vi "Teleop.vi"(10 "Match Info":T1={"Autonomous Elapsed Seconds"=0.0, "TeleOp Elapsed Seconds"=0.0, "Disabled Elapsed Seconds"=0.0, "Visited Autonomous"=FALSE, "Visited TeleOp"=FALSE, "Visited Disabled"=FALSE, "Autonomous Settings"={"Autonomous Style"=enum."Independent", "VI Refnum"=refnum}}, 11 "Call Context":T2) -> ()   [LabVIEW 2014]
doc: "This VI is called for each TeleOp packet received from the DS where the robot is not disabled. It is often used to read from the joysticks and update I/O or to update setpoints for timed control loops. It should complete and return within 20 milliseconds or it may miss DS packets."
uses:
  <vilib>/Rock Robotics/WPI/DriverStation/WPI_DriverStationDerivedRobotMode.ctl
  <vilib>/Rock Robotics/WPI/DriverStation/WPI_DriverStationMatch Info.ctl
  <vilib>/Rock Robotics/WPI/RobotDrive/WPI_RobotDriveGetSetRefNum.vi
  <vilib>/Rock Robotics/WPI/Joystick/WPI_JoystickGetSetRefNum.vi
  <vilib>/Rock Robotics/Network Tables/SD Write Boolean Array.vi
  <vilib>/Rock Robotics/Network Tables/SD Write Numeric Array.vi
  <vilib>/Rock Robotics/Network Tables/SD Read Boolean.vi
  <vilib>/Rock Robotics/Network Tables/SD Read Number.vi
  <vilib>/Rock Robotics/WPI/RobotDrive/WPI_RobotDriveMecanumDrive_Cartesian.vi
panel:
  out "Elevator At Middle":bool
  out "Linear Debug":dbl
  out "Debug":dbl format="%#_13g"
  out "Elevator Up":bool=TRUE
  out "Elevator Down":bool=TRUE
  out "Sample Slider 0":dbl(slide) scale=0.0..5.0
  out "Sample Boolean 1":bool
  out "Sample Boolean 0":bool
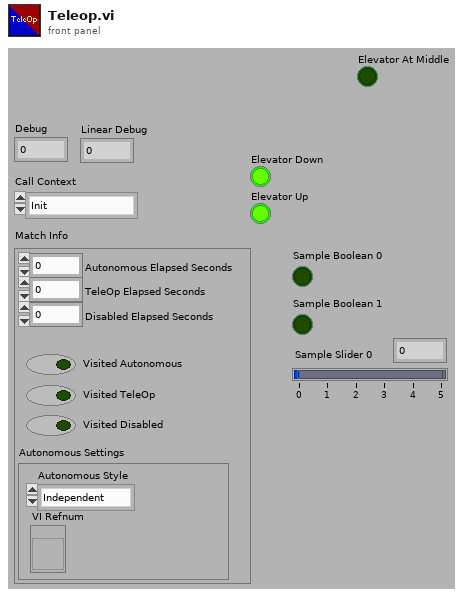
[diagram p1: front panel]
types:
  T1 = typedef "WPI_DriverStationMatch Info.ctl" = cluster{"Autonomous Elapsed Seconds":dbl, "TeleOp Elapsed Seconds":dbl, "Disabled Elapsed Seconds":dbl, "Visited Autonomous":bool, "Visited TeleOp":bool, "Visited Disabled":bool, "Autonomous Settings":cluster{"Autonomous Style":enum16{"Iterative", "Independent"}, "VI Refnum":refnum<vi>}}
  T2 = typedef "WPI_DriverStationDerivedRobotMode.ctl" = enum16{"Init", "Execute", "Stop"}
  T3 = typedef "WPI_RobotDriveDevRef.ctl" = cluster{"DevStatus":errorcluster, "Motors[]":T4[], "Square Inputs":bool, "Max Output":dbl}
  T4 = typedef "WPI_MotorControlDeviceRef.ctl" = cluster{"DeviceStatus":errorcluster, "Type":T5, "PWM":cluster{"Controller":T6, "PWM Channel":T7, "DeadBand":T8}, "CAN":cluster{"Device Number":u8, "Control Mode":T9, "Semaphore":T10, "Max Vout":dbl, "TalonSRX Control Mode":T11}, "Invert":bool, "TransformRef":T12, "InvTransformRef":T12}
  T5 = typedef "WPI_MotorControlType.ctl" = enum16{"PWM", "CAN", "CANTalonSRX"}
  T6 = typedef "FPGA_TypedefDigitalModule.ctl" = enum16{"Controller 1"}
  T7 = typedef "FPGA_DIOPWMChannel.ctl" = enum8{"PWM 0", "PWM 1", "PWM 2", "PWM 3", "PWM 4", "PWM 5", "PWM 6", "PWM 7", "PWM 8", "PWM 9", "PWM MXP 0", "PWM MXP 1", "PWM MXP 2", "PWM MXP 3", "PWM MXP 4", "PWM MXP 5", "PWM MXP 6", "PWM MXP 7", "PWM MXP 8", "PWM MXP 9", "Invalid"}
  T8 = typedef "WPI_PWMDeadband.ctl" = cluster{"Name":string, "maxPositivePwm":i32, "minPositivePwm":i32, "centerPwm":i32, "maxNegativePwm":i32, "minNegativePwm":i32, "angularRange":u16}
  T9 = typedef "WPI_CANJaguar_ControlMode.ctl" = enum8{"Percent VBus", "Current", "Speed", "Position", "Voltage"}
  T10 = typedef "Semaphore RefNum" = refnum<k1>
  T11 = typedef "WPI_CANTalonSRX_APIControlMode.ctl" = enum8{"Percent VBus", "Speed", "Position", "Slave", "Unchanged / Invalid"}
  T12 = typedef "WPI_PWMTransform_ConPane.ctl" = refnum<vi>
  T13 = typedef "WPI_JoystickDevRef.ctl" = cluster{"Device":T14}
  T14 = typedef "WPI_JoystickDeviceEnum.ctl" = enum16{"USB 0", "USB 1", "USB 2", "USB 3", "USB 4", "USB 5"}
  T15 = typedef "WPI_DigitalInputDevRef.ctl" = cluster{"DevStatus":errorcluster, "DIO Channel":T16, "Controller":T6}
  T16 = typedef "FPGA_DIOChannel.ctl" = enum8{"DIO 0", "DIO 1", "DIO 2", "DIO 3", "DIO 4", "DIO 5", "DIO 6", "DIO 7", "DIO 8", "DIO 9", "DIO MXP 0", "DIO MXP 1", "DIO MXP 2", "DIO MXP 3", "DIO MXP 4", "DIO MXP 5", "DIO MXP 6", "DIO MXP 7", "DIO MXP 8", "DIO MXP 9", "DIO MXP 10", "DIO MXP 11", "DIO MXP 12", "DIO MXP 13", "DIO MXP 14", "DIO MXP 15", "Invalid"}
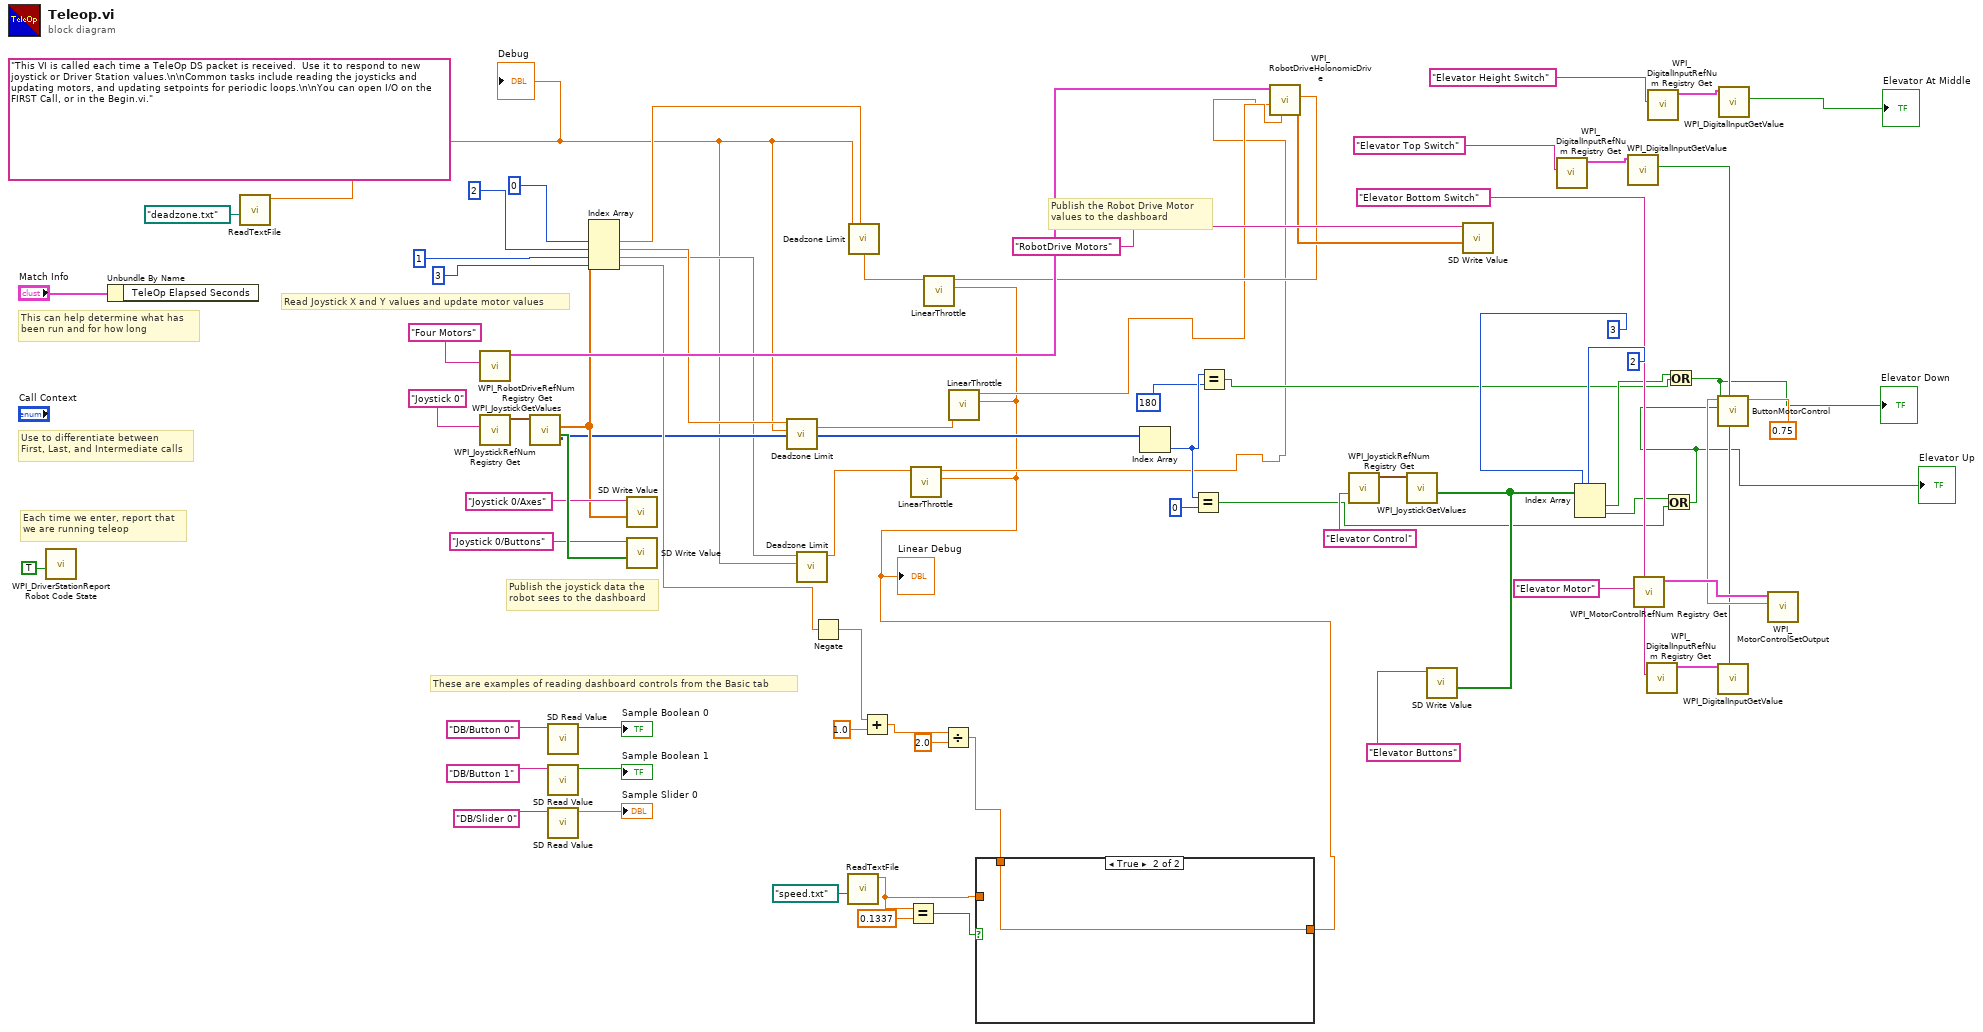
[diagram p0: block diagram]
diagram:
  (unwired) "This VI is called each time a TeleOp DS packet is received.  Use it to respond to new joystick or Driver Station values.\n\nCommon tasks include reading the joysticks and updating motors, and updating setpoints for periodic loops.\n\nYou can open I/O on the FIRST Call, or in the Begin.vi."
  # "These are examples of reading dashboard controls from the Basic tab"
  # "Publish the Robot Drive Motor\nvalues to the dashboard"
  # "Publish the joystick data the\nrobot sees to the dashboard"
  # "Each time we enter, report that\nwe are running teleop"
  # "Use to differentiate between\nFirst, Last, and Intermediate calls"
  # "This can help determine what has\nbeen run and for how long"
  # "Read Joystick X and Y values and update motor values"
  n1 = call <vilib>:"WPI_DriverStationReport Robot Code State.vi"("TeleOp"=TRUE ("Autonomous")) -> ()  [unwired: 10 in, 1 out]
  n2 = Unbundle By Name("Match Info") -> ()  [unwired: 1 out]
  n3 = call "ReadTextFile.vi"("file (use dialog)"=path "/deadzone.txt") -> ("Double"=w7:dbl)  [unwired: 9 in, 1 out]
  "Debug" <- w7
  n4 = call <vilib>:"WPI_RobotDriveRefNum Registry Get.vi"("refnum name"="Four Motors") -> ("RobotDriveDevRef"=w71:T3)  [unwired: 1 in, 9 out]
  n5 = call <vilib>:"WPI_JoystickRefNum Registry Get.vi"("refnum name"="Joystick 0") -> ("JoystickDevRef"=w69:T13)  [unwired: 1 in, 9 out]
  n6 = call <vilib>:"WPI_JoystickGetValues.vi"("JoystickDevRef"=w69) -> ("Buttons"=w67:bool[], "Axes"=w56:dbl[], "POVs"=w28:i16[])  [unwired: 6 in, 2 out]
  n7 = call-poly <vilib>:"SD Read Value.vi"("Name"="DB/Button 0" ("refnum name")) -> ("Boolean"=→"Sample Boolean 0":bool)  [unwired: 8 in, 2 out]
  n8 = call-poly <vilib>:"SD Read Value.vi"("Name"="DB/Button 1" ("refnum name")) -> ("Boolean"=→"Sample Boolean 1":bool)  [unwired: 8 in, 2 out]
  n9 = call-poly <vilib>:"SD Read Value.vi"("Name"="DB/Slider 0" ("refnum name")) -> ("Numeric"=→"Sample Slider 0":dbl)  [unwired: 8 in, 2 out]
  n10 = Index Array(array=w56, index #1=0 ("X"), index #2=2 ("Y"), index #3=1 ("Rotate"), index #4=3 ("throttle")) -> (element #1=w47:dbl, element #2=w46:dbl, element #3=w15:dbl, element #4=w38:dbl)
  n11 = call-poly <vilib>:"SD Write Value.vi"("Numeric Array"=w56, "Name"="Joystick 0/Axes") -> ()  [unwired: 8 in, 2 out]
  n12 = call-poly <vilib>:"SD Write Value.vi"("Boolean Array"=w67, "Name"="Joystick 0/Buttons") -> ()  [unwired: 8 in, 2 out]
  n13 = call "Deadzone Limit.vi"("Limit"=w7, "Input"=w46) -> ("Output"=w41:dbl)  [unwired: 9 in]
  n14 = call "Deadzone Limit.vi"("Limit"=w7, "Input"=w15) -> ("Output"=w40:dbl)  [unwired: 9 in]
  n15 = Negate(x=w38) -> (-x=w39:dbl)
  n16 = call "ReadTextFile.vi"("file (use dialog)"=path "/speed.txt") -> ("Double"=w1:dbl)  [unwired: 9 in, 1 out]
  n17 = call "Deadzone Limit.vi"("Limit"=w7, "Input"=w47) -> ("Output"=w42:dbl)  [unwired: 9 in]
  n18 = Add(x=w39, y=1.0) -> (x+y=w44:dbl)
  n19 = Equal?(x=w1, y=0.1337) -> (x = y?=w4:bool)
  n20 = Divide(x=w44, y=2.0) -> (x/y=w3:dbl)
  n21 = case shown="True" w4 {
    tunnel: w3 -> [_ w75]
    tunnel: [w74 w75] -> w2
    tunnel: w1 -> [w74 _]
    frame False {
    }
    frame True {
    }
  }
  "Linear Debug" <- w2
  n22 = call "LinearThrottle.vi"("Throttle"=w2, "Value"=w40) -> ("Numeric"=w9:dbl)  [unwired: 9 in]
  n23 = call "LinearThrottle.vi"("Throttle"=w2, "Value"=w42) -> ("Numeric"=w37:dbl)  [unwired: 9 in]
  n24 = call "LinearThrottle.vi"("Throttle"=w2, "Value"=w41) -> ("Numeric"=w10:dbl)  [unwired: 9 in]
  n25 = Index Array(array=w28) -> (element=w24:i16)  [unwired: 1 in]
  n26 = Equal?(x=w24, y=i16 0) -> (x = y?=w18:bool)
  n27 = Equal?(x=w24, y=i16 180) -> (x = y?=w19:bool)
  n28 = call-poly <vilib>:"WPI_RobotDriveHolonomicDrive.vi"("Rotation"=w10, "Y"=w9, "X"=w37, "RobotDriveDevRef"=w71) -> ("Motor Values"=w57:dbl[])  [unwired: 5 in, 2 out]
  n29 = call <vilib>:"WPI_JoystickRefNum Registry Get.vi"("refnum name"="Elevator Control") -> ("JoystickDevRef"=w54:T13)  [unwired: 1 in, 9 out]
  n30 = call <vilib>:"WPI_JoystickGetValues.vi"("JoystickDevRef"=w54) -> ("Buttons"=w52:bool[])  [unwired: 6 in, 4 out]
  n31 = call-poly <vilib>:"SD Write Value.vi"("Boolean Array"=w52, "Name"="Elevator Buttons") -> ()  [unwired: 8 in, 2 out]
  n32 = call-poly <vilib>:"SD Write Value.vi"("Numeric Array"=w57, "Name"="RobotDrive Motors") -> ()  [unwired: 8 in, 2 out]
  n33 = call <vilib>:"WPI_DigitalInputRefNum Registry Get.vi"("refnum name"="Elevator Top Switch") -> ("DigitalInputDevRef"=w31:T15)  [unwired: 9 in, 1 out]
  n34 = Index Array(array=w52, index #1=2 ("index"), index #2=3 ("index")) -> (element #1=w21:bool, element #2=w17:bool)
  n35 = call <vilib>:"WPI_DigitalInputGetValue.vi"("DigitalInputDevRef"=w31) -> ("Value"=w30:bool)  [unwired: 8 in, 2 out]
  n36 = call <vilib>:"WPI_MotorControlRefNum Registry Get.vi"("refnum name"="Elevator Motor") -> ("MotorControlDevRef"=w51:T4)  [unwired: 9 in, 1 out]
  n37 = call <vilib>:"WPI_DigitalInputRefNum Registry Get.vi"("refnum name"="Elevator Bottom Switch") -> ("DigitalInputDevRef"=w33:T15)  [unwired: 9 in, 1 out]
  n38 = call <vilib>:"WPI_DigitalInputRefNum Registry Get.vi"("refnum name"="Elevator Height Switch") -> ("DigitalInputDevRef"=w27:T15)  [unwired: 9 in, 1 out]
  n39 = Or(x=w17, y=w18) -> (x .or. y?=w16:bool)
  "Elevator Up" <- w16
  n40 = Or(x=w21, y=w19) -> (x .or. y?=w20:bool)
  "Elevator Down" <- w20
  n41 = call <vilib>:"WPI_DigitalInputGetValue.vi"("DigitalInputDevRef"=w33) -> ("Value"=w32:bool)  [unwired: 8 in, 2 out]
  n42 = call "ButtonMotorControl.vi"("Allow Down"=w32, "Allow Up"=w30, "Down"=w20, "Up"=w16, "Speed"=0.75) -> ("Motor Speed"=w48:dbl)  [unwired: 6 in]
  n43 = call <vilib>:"WPI_DigitalInputGetValue.vi"("DigitalInputDevRef"=w27) -> ("Value"=→"Elevator At Middle":bool)  [unwired: 8 in, 2 out]
  n44 = call <vilib>:"WPI_MotorControlSetOutput.vi"("Output"=w48, "MotorControlDevRef"=w51) -> ()  [unwired: 7 in, 3 out]
